vi "Nodeguard_und_Heartbeat.vi"() -> ()   [LabVIEW 2013]
uses:
  <vilib>/CANopenLib/CANOPEN.llb/CANopen BaudRate.ctl
  <vilib>/CANopenLib/CANOPEN.llb/CANopen Interface Create.vi
  <vilib>/CANopenLib/CANOPEN.llb/CANopen Node Guarding Create.vi
  <vilib>/CANopenLib/CANOPEN.llb/CANopen Node Guarding State Read.vi
  <vilib>/CANopenLib/CANOPEN.llb/CANopen Node Guarding Close.vi
  <vilib>/CANopenLib/CANOPEN.llb/CANopen Interface Close.vi
panel:
  out "error out":errorcluster
  in  "node-ID":u8=2
  out "state":u16(ring) items=["unknown"=1, "bootup"=0, "stopped"=4, "operational"=5, "pre-operational"=127, "connection lost"=128]
  in  "COB-ID (0)":u32=1794
  in  "error in":errorcluster
  in  "Baud Rate 2":T1 items=["1 Mbit/s"=0, "800 kbit/s"=1, "500 kbit/s"=2, "250 kbit/s"=3, "125 kbit/s"=4, "50 kbit/s"=6, "20 kbit/s"=7, "10 kbit/s"=8]
  in  "CANopen Interface 2":u32(ring) items=["CANopen01", "CANopen02", "CANopen03", "CANopen04", "CANopen05", "CANopen06", "CANopen07", "CANopen08", "CANopen09", "CANopen10", "CANopen11", "CANopen12", "CANopen13", "CANopen14", "CANopen15", "CANopen16", "CANopen17", "CANopen18", "CANopen19", "CANopen20", "CANopen21", "CANopen22", "CANopen23", "CANopen24", "CANopen25", "CANopen26", "CANopen27", "CANopen28", "CANopen29", "CANopen30", "CANopen31", "CANopen32"]
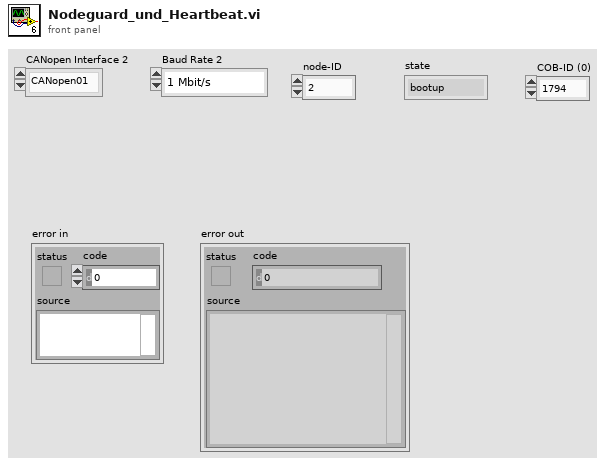
[diagram p1: front panel]
types:
  T1 = typedef "CANopen BaudRate.ctl" = u32
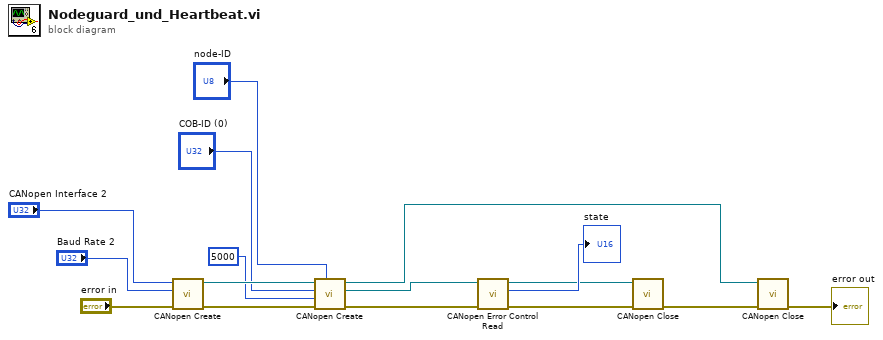
[diagram p0: block diagram]
diagram:
  n1 = call-poly <vilib>:"CANopen Create.vi"("error in (no error)"="error in", "baud rate"="Baud Rate 2", "interface name"="CANopen Interface 2") -> ("error out"=w12:errorcluster, "interface object out"=w13:refnum<k20>)  [unwired: 7 in]
  n2 = call-poly <vilib>:"CANopen Create.vi"("node-ID"="node-ID", "error in (no error)"=w12, "guard time [ms]"=u16 5000, "COB-ID (0)"="COB-ID (0)", "interface object in"=w13) -> ("error out"=w8:errorcluster, "node guarding object out"=w9:refnum<k20>, "interface object out"=w3:refnum<k20>)  [unwired: 4 in]
  n3 = call-poly <vilib>:"CANopen Error Control Read.vi"("error in (no error)"=w8, "node guarding object in"=w9) -> ("error out"=w5:errorcluster, "state"=→"state":u16, "node guarding object out"=w6:refnum<k20>)  [unwired: 6 in, 1 out]
  n4 = call-poly <vilib>:"CANopen Close.vi"("error in (no error)"=w5, "node guarding object in"=w6) -> ("error out"=w4:errorcluster)  [unwired: 9 in]
  n5 = call-poly <vilib>:"CANopen Close.vi"("error in (no error)"=w4, "interface object in"=w3) -> ("error out"=→"error out":errorcluster)  [unwired: 9 in]
